vi "CreateProtectedEvents.vi"(8 "error in (no error)":errorcluster, 11 "XYStage":refnum<class "XYStage.lvclass">) -> (0 "error out":errorcluster, 3 "XYStage out":refnum<class "XYStage.lvclass">)   [LabVIEW 2017, in "XYStage.lvclass"]
doc: "---------------------------------------------------------------\nJKI State Machine Objects™\nhttp://jki.net/state-machine-objects/\nCopyright (C) 2005-2015, JKI <info@jki.net>\nALL RIGHTS RESERVEDJKI State Machine Objects (SMO) 1.0.0.5\nJKI - JKI\nCopyright (c) 2016, JKI"
uses:
  XYStage.lvclass
  XYStage.lvclass/XYStage.ctl
  Typedefs/ProtectedEvents--XYStage.StatusUpdated.ctl
  Typedefs/XYStage.Axis--Enum.ctl
  Typedefs/XYStage.DeviceStatus--Enum.ctl
  Typedefs/ProtectedEvents--XYStage.MoveResultReported.ctl
  Typedefs/Coordinates--Cluster.ctl
  Typedefs/Coordinates.Units--Cluster.ctl
  Typedefs/Coordinates.Counts--Cluster.ctl
  Device/Device.lvclass
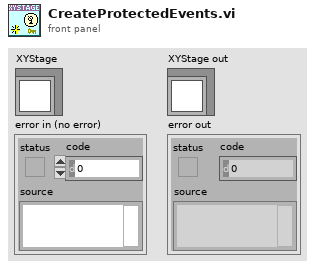
[diagram p1: front panel]
types:
  T1 = typedef "XYStage.lvclass/PrivateData--Ref.ctl" = refnum<data-value>
  T2 = typedef "XYStage.lvclass/ProtectedEvents--XYStage.MoveResultReported.ctl" = cluster{"Result":bool, "Coordinates":T3}
  T3 = typedef "XYStage.lvclass/Coordinates--Cluster.ctl" = cluster{"Units":T4, "Counts":T5}
  T4 = typedef "XYStage.lvclass/Coordinates.Units--Cluster.ctl" = cluster{"X":dbl, "Y":dbl}
  T5 = typedef "XYStage.lvclass/Coordinates.Counts--Cluster.ctl" = cluster{"X":i32, "Y":i32}
  T6 = typedef "XYStage.lvclass/ProtectedEvents--XYStage.StatusUpdated.ctl" = cluster{"Axis":T7, "Position":i32, "IsEnabled":bool, "IsError":bool, "IsMoving":bool, "Status":T8}
  T7 = typedef "XYStage.lvclass/XYStage.Axis--Enum.ctl" = enum16{"X Axis", "Y Axis", "Undefined"}
  T8 = typedef "XYStage.lvclass/XYStage.DeviceStatus--Enum.ctl" = u32
  T9 = typedef "XYStage.lvclass/PrivateData--Cluster.ctl" = cluster{"Configuration":T10, "Public Events":T11, "Protected Events":T12, "Private Events":T13}
  T10 = typedef "XYStage.lvclass/Configuration--Cluster.ctl" = cluster{"Serial Number":string, "X Axis":string, "Y Axis":string, "Real-World Units":string, "Counts per Unit":u32}
  T11 = typedef "XYStage.lvclass/PublicEvents--Cluster.ctl" = cluster{"MoveStarted":refnum<user-event>, "MoveCompleted":refnum<user-event>}
  T12 = typedef "XYStage.lvclass/ProtectedEvents--Cluster.ctl" = cluster{"StatusUpdated":refnum<user-event>, "MoveResultReported":refnum<user-event>}
  T13 = typedef "XYStage.lvclass/PrivateEvents--Cluster.ctl" = cluster{"MoveAbsolute (units)":refnum<user-event>}
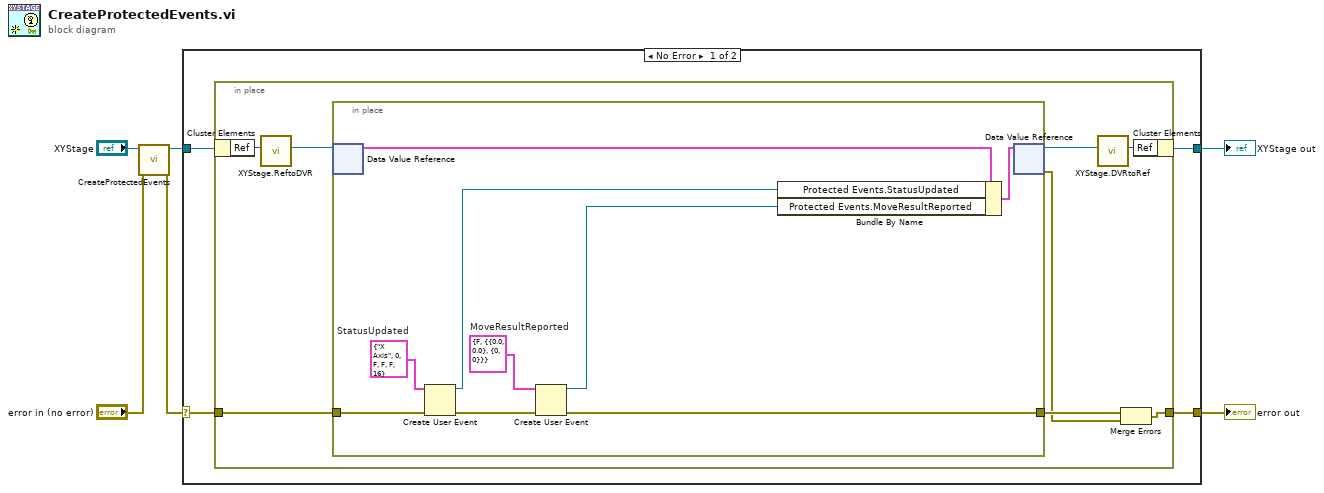
[diagram p0: block diagram]
diagram:
  n1 = call-parent "CreateProtectedEvents.vi"("error in (no error)"="error in (no error)", "SMO"="XYStage") -> ("error out"=w1:errorcluster, "SMO out"=w3:refnum<class "XYStage.lvclass">)  [unwired: 8 in]
  n2 = case shown="No Error" w1 {
    selector: w1 -> [w8 w29]
    tunnel: [w7 w29] -> w5
    tunnel: [w9 w28] -> w6
    tunnel: w3 -> [w10 w28]
    frame No Error {
      n3 = in-place {
        in-place-border: w8 -> [w18]
        in-place-border: [w15] -> w7
        n4 = in-place-cluster #1(w10) -> ("Ref"=w14:u32)
        n5 = call "XYStage.ReftoDVR.vi"("Ref"=w14) -> ("Ref"=w13:T1)  [unwired: 10 in]
        n6 = in-place {
          in-place-border: w18 -> [w26]
          in-place-border: [w21] -> w17
          w19 = T2 {"Result"=FALSE, "Coordinates"={"Units"={"X"=0.0, "Y"=0.0}, "Counts"={"X"=0, "Y"=0}}}  # MoveResultReported
          w24 = T6 {"Axis"=enum."X Axis", "Position"=0, "IsEnabled"=FALSE, "IsError"=FALSE, "IsMoving"=FALSE, "Status"=16}  # StatusUpdated
          n7 = in-place-dvr #2(w13) -> (w25:T9)  [unwired: 1 out]
          n8 = Create User Event(user event datatype=w24, error in=w26) -> (user event=w23:refnum<user-event>, error out=w22:errorcluster)
          n9 = Create User Event(user event datatype=w19, error in=w22) -> (user event=w20:refnum<user-event>, error out=w21:errorcluster)
          n10 = Bundle By Name(cluster=w25, "Protected Events.StatusUpdated"=w23, "Protected Events.MoveResultReported"=w20) -> (w27:T9)
          n11 = in-place-dvr #2(w27) -> (w12:T1, w16:errorcluster)
        }
        n12 = call "XYStage.DVRtoRef.vi"("Ref"=w12) -> ("Ref"=w11:u32)  [unwired: 10 in]
        n13 = Merge Errors(w17, w16) -> (w15:errorcluster)
        n14 = in-place-cluster #1("Ref"=w11) -> (w9:refnum<class "XYStage.lvclass">)
      }
    }
    frame Error {
    }
  }
  "error out" <- w5
  "XYStage out" <- w6
